vi "Write Maximum File Size.vi"(8 "error in (no error)":errorcluster, 10 "Maximum File Size":i64, 11 "TDMS-Actor in":refnum<class "TDMS-Actor.lvclass">=refnum) -> (0 "error out":errorcluster, 3 "TDMS-Actor out":refnum<class "TDMS-Actor.lvclass">)   [LabVIEW 2016, in "BNT_TDMS.lvlib" / "TDMS-Actor.lvclass"]
doc: "Write maxium size for file change to attribute."
uses:
  TDMS-Actor.lvclass
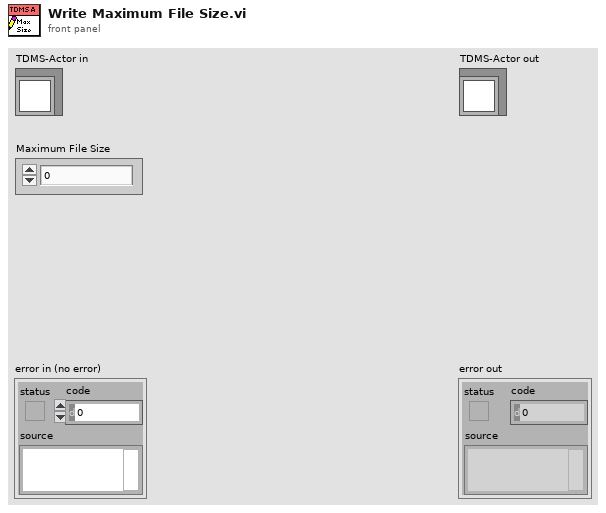
[diagram p1: front panel]
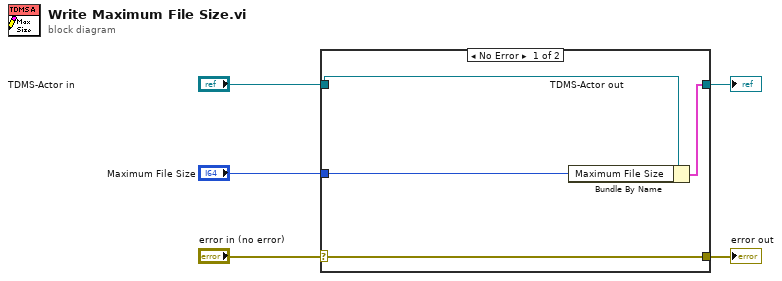
[diagram p0: block diagram]
diagram:
  n1 = case shown="No Error" "error in (no error)" {
    selector: "error in (no error)" -> [w9 w10]
    tunnel: [w9 w10] -> w4
    tunnel: [w7 w11] -> w2
    tunnel: "TDMS-Actor in" -> [w8 w11]
    tunnel: "Maximum File Size" -> [w6 _]
    frame No Error {
      n2 = Bundle By Name(cluster=w8, "Maximum File Size"=w6) -> (w7:cluster{})
    }
    frame Error {
    }
  }
  "error out" <- w4
  "TDMS-Actor out" <- w2
